vi "LBNE_Global .vi"() -> ()   [LabVIEW 2015]
uses:
  E:/P1_ADC_TEST_2017/LabVIEW_1130/LBNE_DLL/LBNE_DLL/bin/Debug/LBNE_DLL.dll
panel:
  out "UDP/I2C":bool=TRUE
  out "LBNE_REF":refnum<k24>
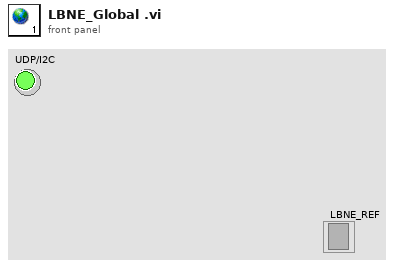
[diagram p1: front panel]
diagram:
